vi "Extract JPEG.vi"(8 "error in (no error)":errorcluster, 11 "Queue in":refnum<queue>) -> (0 "error out":errorcluster, 1 "valid image":bool, 2 "image data":u8[](array[numeric]), 3 "Queue out":refnum<queue>)   [LabVIEW 2013]
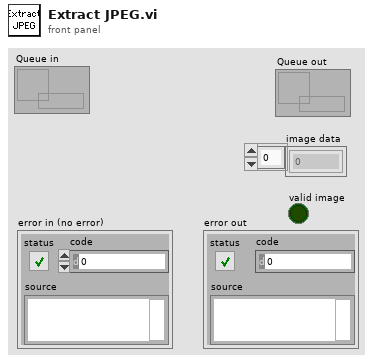
[diagram p1: front panel]
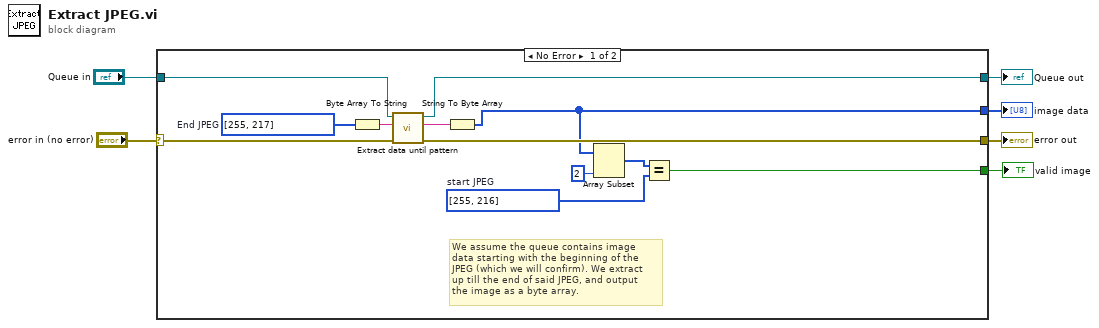
[diagram p0: block diagram]
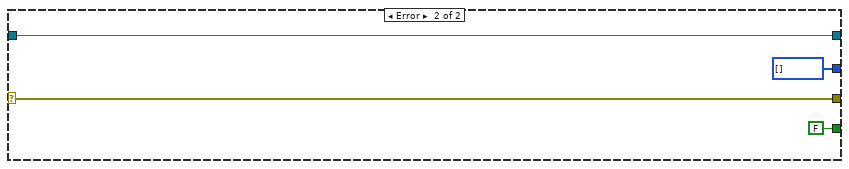
[diagram p2: hidden frame]
diagram:
  n1 = case shown="No Error" "error in (no error)" {
    selector: "error in (no error)" -> [w10 w22]
    tunnel: "Queue in" -> [w18 w21]
    tunnel: [w14 w21] -> w5
    tunnel: [w7 u8[] [] ("unsigned byte array")] -> w4
    tunnel: [w9 w22] -> w3
    tunnel: [w8 FALSE] -> w1
    frame No Error {
      w11 = u8[] [255, 216]  # start JPEG
      w17 = u8[] [255, 217]  # End JPEG
      # "We assume the queue contains image\ndata starting with the beginning of the\nJPEG (which we will confirm). We extract\nup till the end of said JPEG, and output\nthe image as a byte array."
      n2 = Byte Array To String(unsigned byte array=w17) -> (string=w16:string)
      n3 = call "Extract data until pattern.vi"("error in (no error)"=w10, "pattern to match"=w16, "Queue in"=w18) -> ("error out"=w9:errorcluster, "Data until pattern (inclusive)"=w15:string, "Queue out"=w14:refnum<queue>)  [unwired: 6 in]
      n4 = String To Byte Array(string=w15) -> (unsigned byte array=w7:u8[])
      n5 = Array Subset(array=w7, length=2) -> (w12:u8[])  [unwired: 1 in]
      n6 = Equal?(x=w12, y=w11) -> (x = y?=w8:bool)
    }
    frame Error {
    }
  }
  "error out" <- w3
  "Queue out" <- w5
  "image data" <- w4
  "valid image" <- w1
